vi "Update Value Control.vi"(7 "Force update?":bool, 8 "error in (no error)":errorcluster, 9 "Tab Control Ref In":T1, 10 "Tree Control In":refnum<vi>, 11 "Session In":T2) -> (0 "error out":errorcluster, 1 "Units":string, 2 "Tooltip":string, 3 "Session Out":T2)   [LabVIEW 2023]
doc: "The Update Value Control subVI determines the type of the attribute selected, displays the corresponding tab in the tab control, sets the current value of the control, sets the minimum and maximum of the control (for numerics), and disables the control if the attribute is not writables."
uses:
  <vilib>/userdefined/High Color/IMAQdx.ctl
  <vilib>/vision/driver/IMAQdx.llb/IMAQdx Attribute Type.ctl
  <vilib>/vision/driver/NI_Vision_Acquisition_Software.lvlib
  <resource>/objmgr/imaqdx.rc
panel:
  # "Overview: Demonstrates\nRequirements: Vision Acquisition Software\nInstructions: Run the VI"
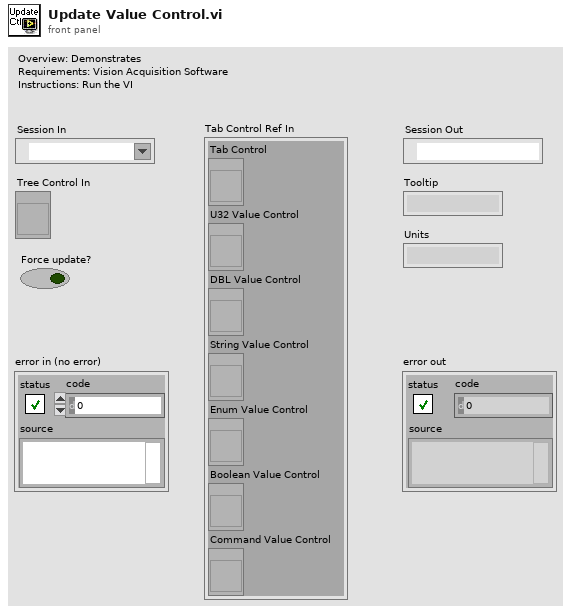
[diagram p1: front panel]
types:
  T1 = cluster{"Tab Control":refnum<vi>, "U32 Value Control":refnum<vi>, "DBL Value Control":refnum<vi>, "String Value Control":refnum<vi>, "Enum Value Control":refnum<vi>, "Boolean Value Control":refnum<vi>, "Command Value Control":refnum<vi>}
  T2 = typedef "IMAQdx.ctl" = refnum<k21>
  T3 = enum8{"Enabled", "Disabled", "Disabled and Grayed Out"}
  T4 = typedef "NI_Vision_Acquisition_Software.lvlib/IMAQdx Attribute Type.ctl" = enum32{"U32", "I64", "DBL", "String", "Enum", "Bool", "Command"}
  T5 = enum32{"U32", "DBL", "String", "Enum", "Bool", "Command"}
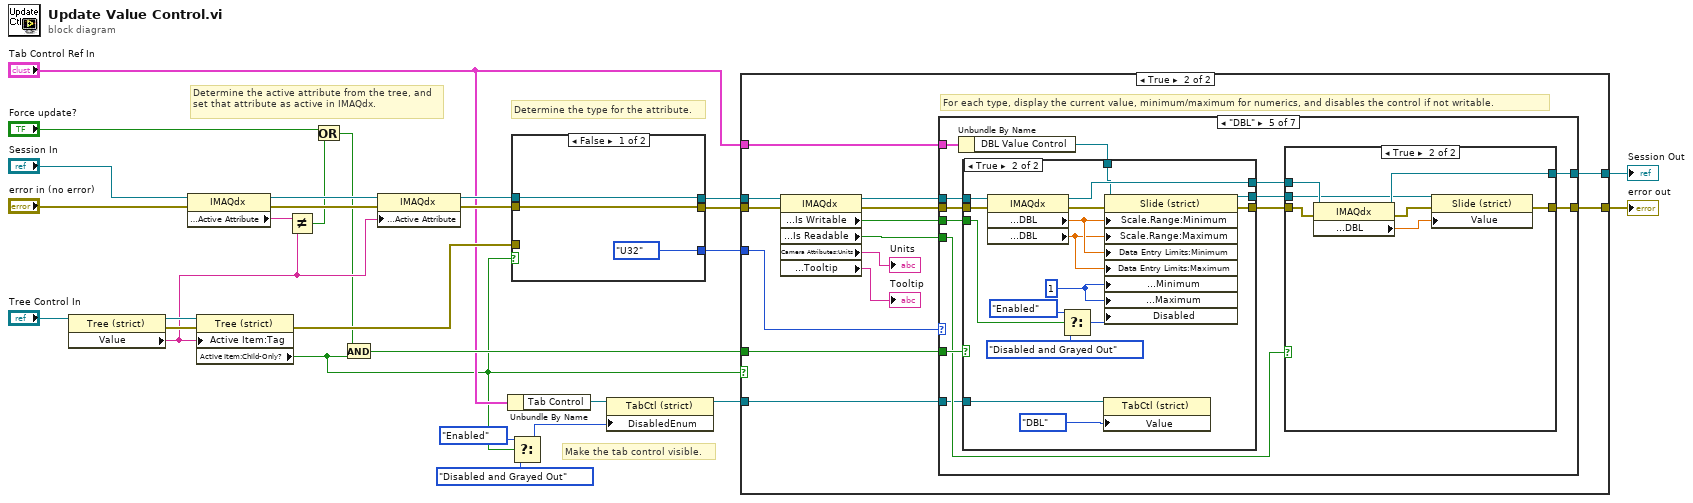
[diagram p0: block diagram]
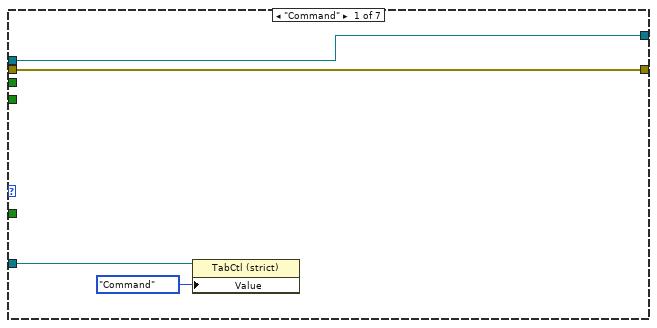
[diagram p3: hidden frame]
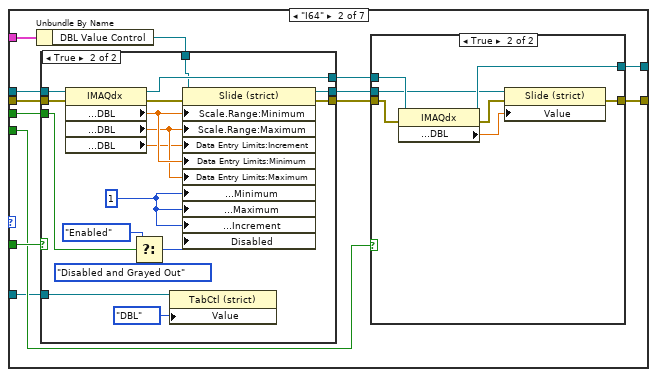
[diagram p4: hidden frame]
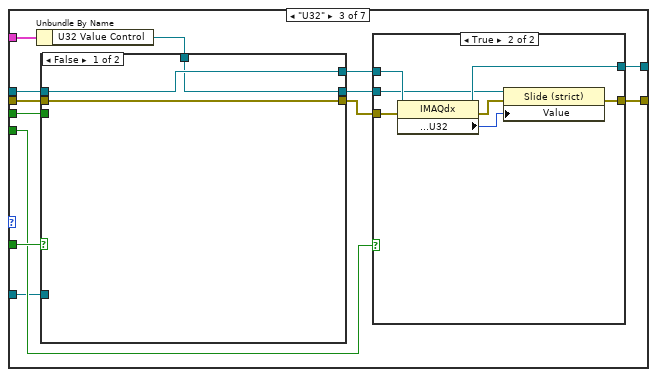
[diagram p7: hidden frame]
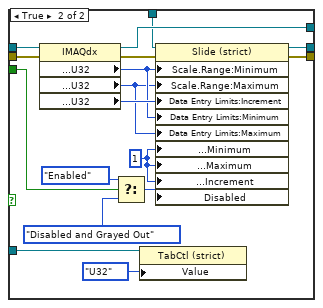
[diagram p9: hidden frame]
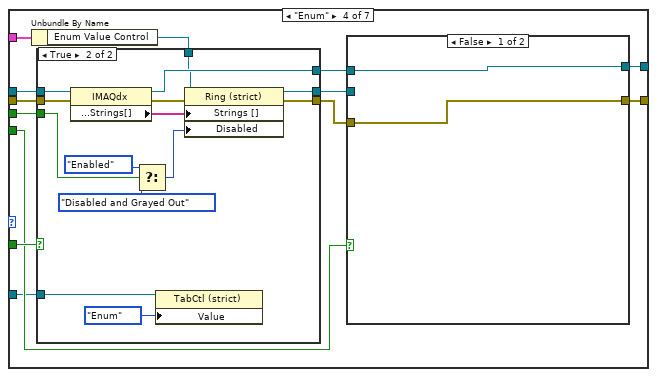
[diagram p10: hidden frame]
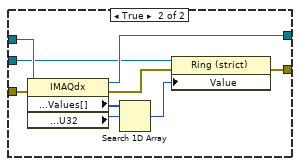
[diagram p11: hidden frame]
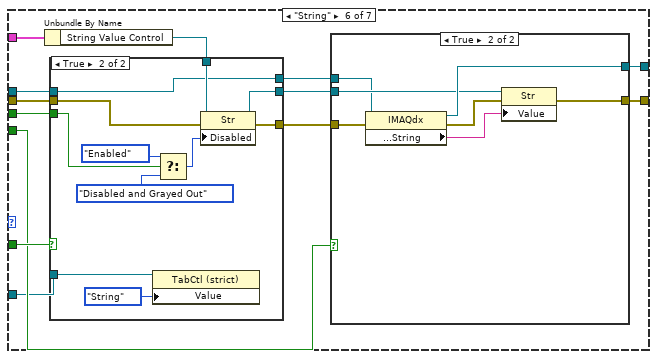
[diagram p15: hidden frame]
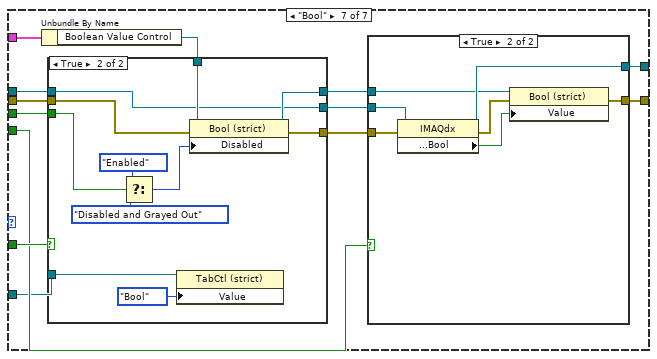
[diagram p18: hidden frame]
diagram:
  # "Make the tab control visible."
  # "Determine the type for the attribute."
  # "Determine the active attribute from the tree, and set that attribute as active in IMAQdx."
  n1 = property class="Tree (strict)"(reference="Tree Control In") -> (reference out=w14:refnum<vi>, error out=w13:errorcluster, "Value"=w12:string)  [unwired: 1 in]
  n2 = property class="IMAQdx"(reference="Session In", error in="error in (no error)") -> (reference out=w27:T2, error out=w26:errorcluster, "Camera Attributes:Active Attribute"=w28:string)
  n3 = property class="Tree (strict)"(reference=w14, error in=w13, "Active Item:Tag"=w12) -> (error out=w19:errorcluster, "Active Item:Child-Only?"=w2:bool)  [unwired: 1 out]
  n4 = Not Equal?(x=w28, y=w12) -> (x != y?=w7:bool)
  n5 = Or(x="Force update?", y=w7) -> (x .or. y?=w5:bool)
  n6 = And(x=w5, y=w2) -> (x .and. y?=w20:bool)
  n7 = property class="IMAQdx"(reference=w27, error in=w26, "Camera Attributes:Active Attribute"=w12) -> (reference out=w25:T2, error out=w24:errorcluster)
  n8 = Unbundle By Name("Tab Control Ref In") -> ("Tab Control"=w10:refnum<vi>)
  n9 = case shown="False" w2 {
    tunnel: w25 -> [w31 w38]
    tunnel: [w31 w35] -> w22
    tunnel: [IMAQdx_Attribute_Type."U32" ("Attribute Type") w34] -> w21
    tunnel: w24 -> [w29 w33]
    tunnel: [w29 w32] -> w23
    tunnel: w19 -> [_ _]
    frame False {
    }
    frame True {
      n10 = property class="IMAQdx"(reference=w38, error in=w33) -> (reference out=w35:T2, error out=w32:errorcluster, "Camera Attributes:Type"=w37:u32)
      n11 = Type Cast(type=IMAQdx_Attribute_Type."U32" ("Attribute Type"), x=w37) -> (*(type *) &x=w34:T4)
    }
  }
  n12 = Select(t=T3."Enabled" ("Disabled"), s=w2, f=T3."Disabled and Grayed Out" ("Disabled")) -> (s? t:f=w1:T3)
  n13 = property class="TabCtl (strict)"(reference=w10, "DisabledEnum"=w1) -> (reference out=w8:refnum<vi>)  [unwired: 1 in, 1 out]
  n14 = case shown="True" w2 {
    tunnel: w23 -> [w40 w53]
    tunnel: [w40 w46] -> w15
    tunnel: w22 -> [w39 w54]
    tunnel: w21 -> [_ w51]
    tunnel: w20 -> [_ w41]
    tunnel: [w39 w45] -> w16
    tunnel: "Tab Control Ref In" -> [_ w44]
    tunnel: w8 -> [_ w43]
    frame False {
    }
    frame True {
      # "For each type, display the current value, minimum/maximum for numerics, and disables the control if not writable."
      n15 = property class="IMAQdx"(reference=w54, error in=w53) -> (reference out=w48:T2, error out=w47:errorcluster, "Camera Attributes:Is Writable"=w50:bool, "Camera Attributes:Is Readable"=w49:bool, "Camera Attributes:Units"=→"Units":string, "Camera Attributes:Tooltip"=→"Tooltip":string)
      n16 = case shown="\"DBL\"" w51 {
        tunnel: w50 -> [_ w68 w110 w152 w193 w234 w270]
        tunnel: w49 -> [_ w67 w109 w151 w192 w233 w269]
        tunnel: w48 -> [w57 w71 w113 w155 w196 w237 w273]
        tunnel: w47 -> [w58 w70 w112 w154 w195 w236 w272]
        tunnel: w41 -> [_ w69 w111 w153 w194 w235 w271]
        tunnel: [w58 w64 w106 w149 w189 w231 w267] -> w46
        tunnel: [w57 w63 w105 w148 w188 w230 w266] -> w45
        tunnel: w44 -> [_ w61 w102 w145 w187 w228 w264]
        tunnel: w43 -> [w56 w62 w103 w146 w185 w229 w265]
        frame "Command" {
          n17 = property class="TabCtl (strict)"(reference=w56, "Value"=T5."Command" ("Tab Control")) -> ()  [unwired: 1 in, 2 out]
        }
        frame "I64" {
          n18 = Unbundle By Name(w61) -> ("DBL Value Control"=w60:refnum<vi>)
          n19 = case shown="True" w69 {
            tunnel: w71 -> [w83 w100]
            tunnel: w70 -> [w82 w99]
            tunnel: [w83 w95] -> w66
            tunnel: [w82 w91] -> w65
            tunnel: w68 -> [_ w98]
            tunnel: w62 -> [_ w97]
            tunnel: w60 -> [w81 w93]
            tunnel: [w81 w92] -> w59
            frame False {
            }
            frame True {
              w87 = u8 1 ("Out Of Range Action:Maximum")
              n20 = property class="IMAQdx"(reference=w100, error in=w99) -> (reference out=w95:T2, error out=w94:errorcluster, "Camera Attributes:Minimum:DBL"=w89:dbl, "Camera Attributes:Maximum:DBL"=w88:dbl, "Camera Attributes:Increment:DBL"=w86:dbl)
              n21 = Select(t=T3."Enabled" ("Disabled"), s=w98, f=T3."Disabled and Grayed Out" ("Disabled")) -> (s? t:f=w90:T3)
              n22 = property class="TabCtl (strict)"(reference=w97, "Value"=T5."DBL" ("Tab Control")) -> ()  [unwired: 1 in, 2 out]
              n23 = property class="Slide (strict)"(reference=w93, error in=w94, "Scale.Range:Minimum"=w89, "Scale.Range:Maximum"=w88, "Data Entry Limits:Increment"=w86, "Data Entry Limits:Minimum"=w89, "Data Entry Limits:Maximum"=w88, "Response to Value Outside Limits:Minimum"=w87, "Response to Value Outside Limits:Maximum"=w87, "Response to Value Outside Limits:Increment"=w87, "Disabled"=w90) -> (reference out=w92:refnum<vi>, error out=w91:errorcluster)
            }
          }
          n24 = case shown="True" w67 {
            tunnel: w66 -> [w73 w80]
            tunnel: w65 -> [w72 w79]
            tunnel: [w73 w77] -> w63
            tunnel: [w72 w78] -> w64
            tunnel: w59 -> [_ w75]
            frame False {
            }
            frame True {
              n25 = property class="IMAQdx"(reference=w80, error in=w79) -> (reference out=w77:T2, error out=w76:errorcluster, "Camera Attributes:Value:DBL"=w74:dbl)
              n26 = property class="Slide (strict)"(reference=w75, error in=w76, "Value"=w74) -> (error out=w78:errorcluster)  [unwired: 1 out]
            }
          }
        }
        frame "U32" {
          n27 = Unbundle By Name(w102) -> ("U32 Value Control"=w101:refnum<vi>)
          n28 = case shown="False" w111 {
            tunnel: w113 -> [w125 w142]
            tunnel: w112 -> [w124 w141]
            tunnel: [w125 w138] -> w108
            tunnel: [w124 w136] -> w107
            tunnel: w110 -> [_ w140]
            tunnel: [w123 w135] -> w104
            tunnel: w103 -> [_ w134]
            tunnel: w101 -> [w123 w132]
            frame False {
            }
            frame True {
              w131 = u8 1 ("Out Of Range Action:Maximum")
              n29 = property class="IMAQdx"(reference=w142, error in=w141) -> (reference out=w138:T2, error out=w139:errorcluster, "Camera Attributes:Minimum:U32"=w129:u32, "Camera Attributes:Maximum:U32"=w128:u32, "Camera Attributes:Increment:U32"=w130:u32)
              n30 = Select(t=T3."Enabled" ("Disabled"), s=w140, f=T3."Disabled and Grayed Out" ("Disabled")) -> (s? t:f=w137:T3)
              n31 = property class="TabCtl (strict)"(reference=w134, "Value"=T5."U32" ("Tab Control")) -> ()  [unwired: 1 in, 2 out]
              n32 = property class="Slide (strict)"(reference=w132, error in=w139, "Scale.Range:Minimum"=w129, "Scale.Range:Maximum"=w128, "Data Entry Limits:Increment"=w130, "Data Entry Limits:Minimum"=w129, "Data Entry Limits:Maximum"=w128, "Response to Value Outside Limits:Minimum"=w131, "Response to Value Outside Limits:Maximum"=w131, "Response to Value Outside Limits:Increment"=w131, "Disabled"=w137) -> (reference out=w135:refnum<vi>, error out=w136:errorcluster)
            }
          }
          n33 = case shown="True" w109 {
            tunnel: w108 -> [w115 w122]
            tunnel: w107 -> [w114 w121]
            tunnel: [w115 w120] -> w105
            tunnel: [w114 w116] -> w106
            tunnel: w104 -> [_ w117]
            frame False {
            }
            frame True {
              n34 = property class="IMAQdx"(reference=w122, error in=w121) -> (reference out=w120:T2, error out=w119:errorcluster, "Camera Attributes:Value:U32"=w118:u32)
              n35 = property class="Slide (strict)"(reference=w117, error in=w119, "Value"=w118) -> (error out=w116:errorcluster)  [unwired: 1 out]
            }
          }
        }
        frame "Enum" {
          n36 = Unbundle By Name(w145) -> ("Enum Value Control"=w144:refnum<vi>)
          n37 = case shown="True" w153 {
            tunnel: w155 -> [w169 w183]
            tunnel: w154 -> [w168 w182]
            tunnel: [w169 w180] -> w150
            tunnel: [w168 w178] -> w143
            tunnel: w152 -> [_ w181]
            tunnel: [w167 w177] -> w147
            tunnel: w146 -> [_ w174]
            tunnel: w144 -> [w167 w172]
            frame False {
            }
            frame True {
              n38 = property class="IMAQdx"(reference=w183, error in=w182) -> (reference out=w180:T2, error out=w179:errorcluster, "Camera Attributes:Enum:Strings[]"=w175:string[])
              n39 = Select(t=T3."Enabled" ("Disabled"), s=w181, f=T3."Disabled and Grayed Out" ("Disabled")) -> (s? t:f=w176:T3)
              n40 = property class="TabCtl (strict)"(reference=w174, "Value"=T5."Enum" ("Tab Control")) -> ()  [unwired: 1 in, 2 out]
              n41 = property class="Ring (strict)"(reference=w172, error in=w179, "Strings []"=w175, "Disabled"=w176) -> (reference out=w177:refnum<vi>, error out=w178:errorcluster)
            }
          }
          n42 = case shown="False" w151 {
            tunnel: w150 -> [w157 w166]
            tunnel: [w157 w161] -> w148
            tunnel: [w156 w163] -> w149
            tunnel: w147 -> [_ w160]
            tunnel: w143 -> [w156 w158]
            frame False {
            }
            frame True {
              n43 = property class="IMAQdx"(reference=w166, error in=w158) -> (reference out=w161:T2, error out=w159:errorcluster, "Camera Attributes:Enum:Values[]"=w165:u32[], "Camera Attributes:Value:U32"=w164:u32)
              n44 = Search 1D Array(1D array=w165, element=w164) -> (index of element=w162:i32)  [unwired: 1 out]
              n45 = property class="Ring (strict)"(reference=w160, error in=w159, "Value"=w162) -> (error out=w163:errorcluster)  [unwired: 1 out]
            }
          }
        }
        frame "DBL" {
          n46 = Unbundle By Name(w187) -> ("DBL Value Control"=w186:refnum<vi>)
          n47 = case shown="True" w194 {
            tunnel: w196 -> [w208 w224]
            tunnel: w195 -> [w207 w223]
            tunnel: [w208 w222] -> w191
            tunnel: [w207 w217] -> w190
            tunnel: w193 -> [_ w209]
            tunnel: w186 -> [w206 w220]
            tunnel: [w206 w219] -> w184
            tunnel: w185 -> [_ w216]
            frame False {
            }
            frame True {
              w210 = u8 1 ("Out Of Range Action:Minimum")
              n48 = property class="IMAQdx"(reference=w224, error in=w223) -> (reference out=w222:T2, error out=w221:errorcluster, "Camera Attributes:Minimum:DBL"=w214:dbl, "Camera Attributes:Maximum:DBL"=w213:dbl)
              n49 = Select(t=T3."Enabled" ("Disabled"), s=w209, f=T3."Disabled and Grayed Out" ("Disabled")) -> (s? t:f=w218:T3)
              n50 = property class="TabCtl (strict)"(reference=w216, "Value"=T5."DBL" ("Tab Control")) -> ()  [unwired: 1 in, 2 out]
              n51 = property class="Slide (strict)"(reference=w220, error in=w221, "Scale.Range:Minimum"=w214, "Scale.Range:Maximum"=w213, "Data Entry Limits:Minimum"=w214, "Data Entry Limits:Maximum"=w213, "Response to Value Outside Limits:Minimum"=w210, "Response to Value Outside Limits:Maximum"=w210, "Disabled"=w218) -> (reference out=w219:refnum<vi>, error out=w217:errorcluster)
            }
          }
          n52 = case shown="True" w192 {
            tunnel: w191 -> [w198 w205]
            tunnel: w190 -> [w197 w204]
            tunnel: [w198 w203] -> w188
            tunnel: [w197 w201] -> w189
            tunnel: w184 -> [_ w200]
            frame False {
            }
            frame True {
              n53 = property class="IMAQdx"(reference=w205, error in=w204) -> (reference out=w203:T2, error out=w202:errorcluster, "Camera Attributes:Value:DBL"=w199:dbl)
              n54 = property class="Slide (strict)"(reference=w200, error in=w202, "Value"=w199) -> (error out=w201:errorcluster)  [unwired: 1 out]
            }
          }
        }
        frame "String" {
          n55 = Unbundle By Name(w228) -> ("String Value Control"=w227:refnum<vi>)
          n56 = case shown="True" w235 {
            tunnel: w237 -> [w247 w252]
            tunnel: w236 -> [w249 w256]
            tunnel: [w249 w255] -> w232
            tunnel: w234 -> [_ w260]
            tunnel: w229 -> [_ w259]
            tunnel: w227 -> [w248 w257]
            tunnel: [w248 w253] -> w226
            tunnel: [w247 w252] -> w225
            frame False {
            }
            frame True {
              n57 = property class="TabCtl (strict)"(reference=w259, "Value"=T5."String" ("Tab Control")) -> ()  [unwired: 1 in, 2 out]
              n58 = Select(t=T3."Enabled" ("Disabled"), s=w260, f=T3."Disabled and Grayed Out" ("Disabled")) -> (s? t:f=w254:T3)
              n59 = property class="Str"(reference=w257, error in=w256, "Disabled"=w254) -> (reference out=w253:refnum<vi>, error out=w255:errorcluster)
            }
          }
          n60 = case shown="True" w233 {
            tunnel: w232 -> [w239 w246]
            tunnel: [w238 w245] -> w230
            tunnel: [w239 w243] -> w231
            tunnel: w226 -> [_ w241]
            tunnel: w225 -> [w238 w240]
            frame False {
            }
            frame True {
              n61 = property class="IMAQdx"(reference=w240, error in=w246) -> (reference out=w245:T2, error out=w244:errorcluster, "Camera Attributes:Value:String"=w242:string)
              n62 = property class="Str"(reference=w241, error in=w244, "Value"=w242) -> (error out=w243:errorcluster)  [unwired: 1 out]
            }
          }
        }
        frame "Bool" {
          n63 = Unbundle By Name(w264) -> ("Boolean Value Control"=w263:refnum<vi>)
          n64 = case shown="True" w271 {
            tunnel: w273 -> [w283 w288]
            tunnel: w272 -> [w285 w291]
            tunnel: [w285 w290] -> w268
            tunnel: w270 -> [_ w296]
            tunnel: w265 -> [_ w295]
            tunnel: w263 -> [w284 w293]
            tunnel: [w284 w292] -> w262
            tunnel: [w283 w288] -> w261
            frame False {
            }
            frame True {
              n65 = Select(t=T3."Enabled" ("Disabled"), s=w296, f=T3."Disabled and Grayed Out" ("Disabled")) -> (s? t:f=w289:T3)
              n66 = property class="TabCtl (strict)"(reference=w295, "Value"=T5."Bool" ("Tab Control")) -> ()  [unwired: 1 in, 2 out]
              n67 = property class="Bool (strict)"(reference=w293, error in=w291, "Disabled"=w289) -> (reference out=w292:refnum<vi>, error out=w290:errorcluster)
            }
          }
          n68 = case shown="True" w269 {
            tunnel: w268 -> [w275 w282]
            tunnel: [w274 w281] -> w266
            tunnel: [w275 w279] -> w267
            tunnel: w262 -> [_ w277]
            tunnel: w261 -> [w274 w276]
            frame False {
            }
            frame True {
              n69 = property class="IMAQdx"(reference=w276, error in=w282) -> (reference out=w281:T2, error out=w280:errorcluster, "Camera Attributes:Value:Bool"=w278:bool)
              n70 = property class="Bool (strict)"(reference=w277, error in=w280, "Value"=w278) -> (error out=w279:errorcluster)  [unwired: 1 out]
            }
          }
        }
      }
    }
  }
  "Session Out" <- w16
  "error out" <- w15
